vi "ge_SortFilterArray.vi"(3 "V Ranges":u16[](array[numeric])) -> (1 "Array":u16[](array[numeric]))   [LabVIEW 2012]
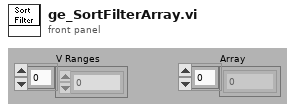
[diagram p1: front panel]
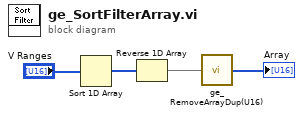
[diagram p0: block diagram]
diagram:
  n1 = Sort 1D Array(array="V Ranges") -> (sorted array=w3:u16[])
  n2 = Reverse 1D Array(array=w3) -> (reversed array=w2:u16[])
  n3 = call "ge_RemoveArrayDup(U16).vi"("Input Array"=w2) -> ("Output Array"=→"Array":u16[])  [unwired: 4 in]
